vi "Proceed.vi"(7 "component is ready (Y)":bool=TRUE, 8 "error in (no error)":errorcluster, 10 "ProceedMessage":refnum<class "ProceedMessage.lvclass">, 11 "DAQOrcaFlash in":refnum<class "DAQOrcaFlash.lvclass">) -> (0 "error out":errorcluster, 2 "all observers are ready?":bool, 3 "DAQOrcaFlash out":refnum<class "DAQOrcaFlash.lvclass">)   [LabVIEW 2012, in "DAQOrcaFlash.lvclass"]
uses:
  DAQOrcaFlash.lvclass
  <vilib>/Distrio/Murmex/ProceedMessage/ProceedMessage.lvclass
  DAQOrcaFlash.lvclass/DAQOrcaFlash.ctl
  <vilib>/Distrio/Murmex/Murmex/Murmex.lvclass
panel:
  # "This method is called when the PROCEED\ntrigger is sent. \n\nOverride this method when your component needs to\nrespond to this trigger. \n\nCall parent for proper implementation"
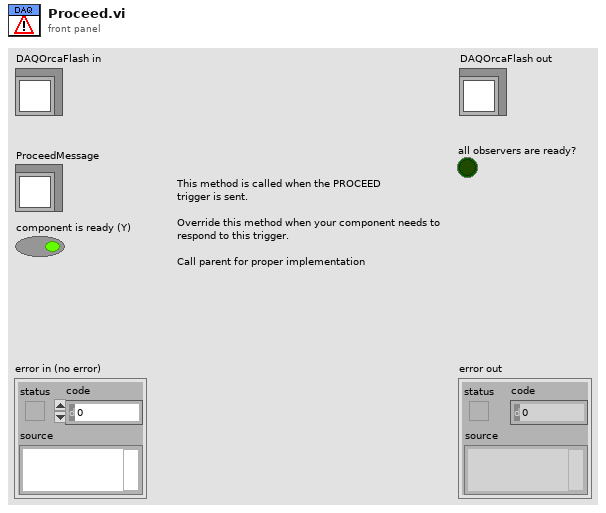
[diagram p1: front panel]
types:
  T1 = typedef "DAQOrcaFlash.lvclass/imaging_mode.ctl" = enum16{"focus mode", "single sweep"}
  T2 = typedef "IMAQ Image.ctl" = refnum<image>
  T3 = cluster{"width":u32, "height":u32, "datatype":u32}
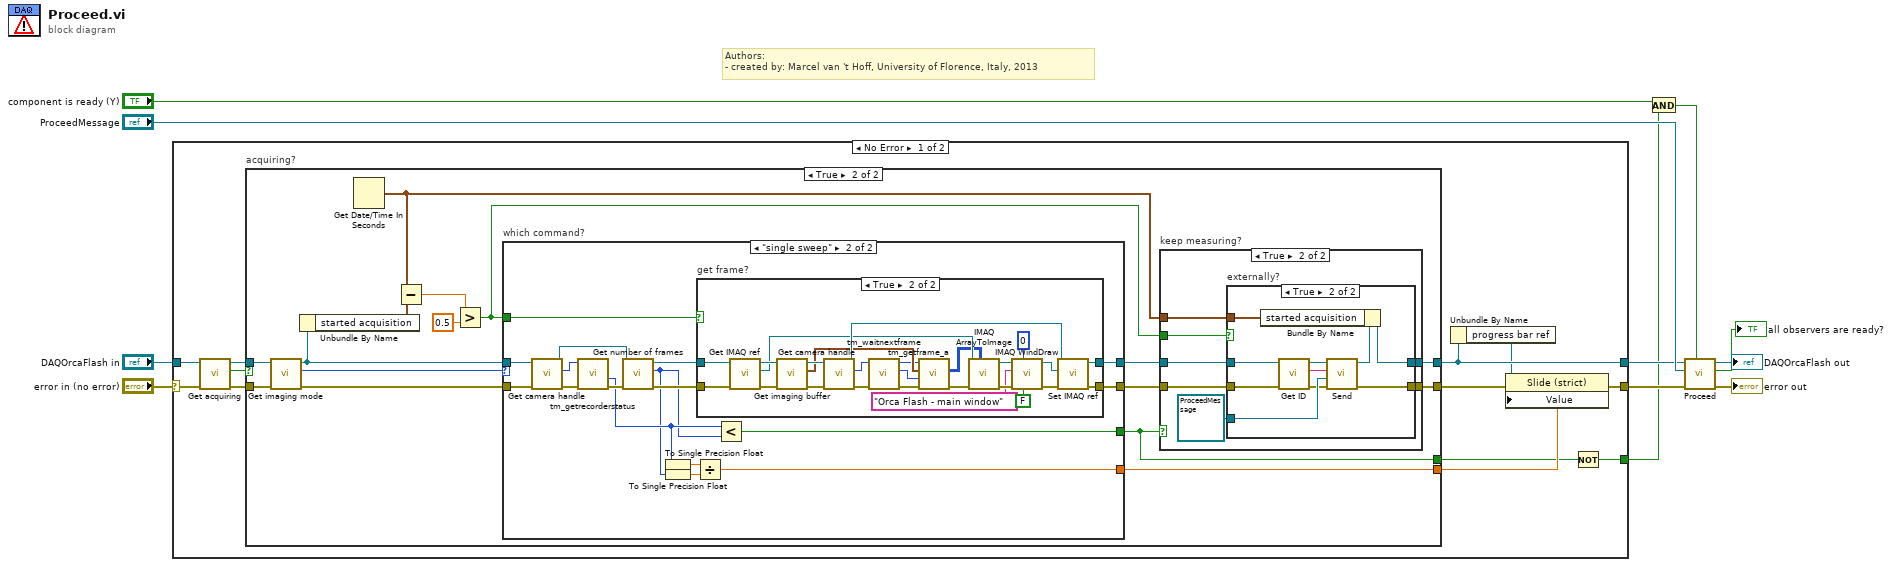
[diagram p0: block diagram]
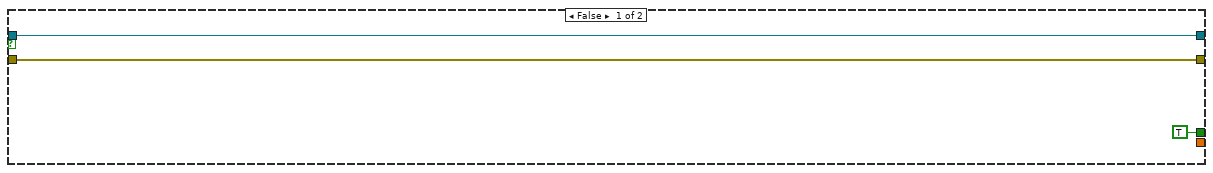
[diagram p2: hidden frame]
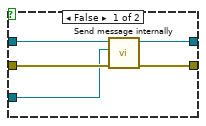
[diagram p4: hidden frame]
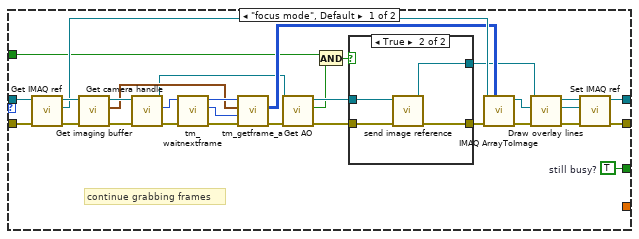
[diagram p5: hidden frame]
diagram:
  # "Authors: \n- created by: Marcel van 't Hoff, University of Florence, Italy, 2013"
  n1 = case shown="No Error" "error in (no error)" {
    selector: "error in (no error)" -> [w21 w149]
    tunnel: [w15 w149] -> w6
    tunnel: [w18 w148] -> w5
    tunnel: "DAQOrcaFlash in" -> [w23 w148]
    tunnel: [w12 _] -> w3
    frame No Error {
      n2 = call "Get acquiring.vi"("error in (no error)"=w21, "DAQMH121119OrcaFlash in"=w23) -> ("error out"=w20:errorcluster, "is acquiring?"=w19:bool, "DAQMH121119OrcaFlash out"=w22:refnum<class "DAQOrcaFlash.lvclass">)  [unwired: 7 in]
      n3 = case "acquiring?" shown="True" w19 {
        tunnel: [w25 w34] -> w14
        tunnel: [w26 w35] -> w18
        tunnel: w22 -> [w26 w40]
        tunnel: w20 -> [w25 w39]
        tunnel: [_ w38] -> w16
        tunnel: [TRUE ("proceed?") w27] -> w13
        frame False {
        }
        frame True {
          n4 = call "Get imaging mode.vi"("error in (no error)"=w39, "DAQMH121119OrcaFlash in"=w40) -> ("error out"=w42:errorcluster, "imaging mode"=w41:T1, "DAQMH121119OrcaFlash out"=w30:refnum<class "DAQOrcaFlash.lvclass">)  [unwired: 7 in]
          n5 = Unbundle By Name(w30) -> ("started acquisition"=w31:timestamp)
          n6 = Get Date/Time In Seconds() -> (seconds since 1Jan1904=w29:timestamp)
          n7 = Subtract(x=w29, y=w31) -> (x-y=w32:dbl)
          n8 = Greater?(x=w32, y=0.5) -> (0:w28:bool)
          n9 = case "which command?" shown="\"single sweep\"" w41 {
            tunnel: w42 -> [w96 w120]
            tunnel: w30 -> [w97 w118]
            tunnel: [w95 w108] -> w37
            tunnel: [w94 w109] -> w36
            tunnel: [_ w110] -> w38
            tunnel: [w93 w104] -> w27
            tunnel: w28 -> [w74 w107]
            frame "focus mode", Default {
              w93 = TRUE  # still busy?
              # "continue grabbing frames"
              n10 = call "Get IMAQ ref.vi"("error in (no error)"=w96, "DAQMH121119OrcaFlash in"=w97) -> ("error out"=w88:errorcluster, "IMAQ reference"=w82:T2, "DAQMH121119OrcaFlash out"=w90:refnum<class "DAQOrcaFlash.lvclass">)  [unwired: 7 in]
              n11 = call "Get imaging buffer.vi"("error in (no error)"=w88, "DAQMH121119OrcaFlash in"=w90) -> ("error out"=w87:errorcluster, "imaging buffer"=w84:T3, "DAQMH121119OrcaFlash out"=w89:refnum<class "DAQOrcaFlash.lvclass">)  [unwired: 5 in, 2 out]
              n12 = call "Get camera handle.vi"("error in (no error)"=w87, "DAQMH121119OrcaFlash in"=w89) -> ("error out"=w91:errorcluster, "cam handle"=w92:u32, "DAQMH121119OrcaFlash out"=w77:refnum<class "DAQOrcaFlash.lvclass">)  [unwired: 7 in]
              n13 = call <userlib>:"tm_waitnextframe.vi"("error in (no error)"=w91, "Handle in"=w92) -> ("error out"=w86:errorcluster, "Frame Index"=w83:i32, "Handle out"=w85:u32)  [unwired: 6 in, 1 out]
              n14 = call <userlib>:"tm_getframe_a.vi"("error in (no error)"=w86, "Frame Index"=w83, "Buffer"=w84, "Handle in"=w85) -> ("error out"=w79:errorcluster, "Data 16"=w80:u16[][])  [unwired: 3 in, 3 out]
              n15 = call-dynamic "Get AO.vi"("error in (no error)"=w79, "DAQOrcaFlash in"=w77) -> ("error out"=w78:errorcluster, "AO"=w75:bool, "DAQOrcaFlash out"=w76:refnum<class "DAQOrcaFlash.lvclass">)  [unwired: 7 in]
              n16 = And(x=w74, y=w75) -> (x .and. y?=w73:bool)
              n17 = case shown="True" w73 {
                tunnel: [w99 w101] -> w81
                tunnel: w78 -> [w99 w103]
                tunnel: w76 -> [w98 w102]
                tunnel: [w98 w100] -> w67
                frame False {
                }
                frame True {
                  n18 = call-dynamic "send image reference.vi"("error in (no error)"=w103, "DAQOrcaFlash in"=w102) -> ("error out"=w101:errorcluster, "DAQOrcaFlash out"=w100:refnum<class "DAQOrcaFlash.lvclass">)  [unwired: 8 in]
                }
              }
              n19 = call "IMAQ ArrayToImage"("Image Pixels (U16)"=w80, "error in (no error)"=w81, "Image"=w82) -> ("error out"=w72:errorcluster, "Image Out"=w70:T2)  [unwired: 7 in]
              n20 = call "Draw overlay lines.vi"("error in (no error)"=w72, "IMAQ reference"=w70, "DAQOrcaFlash in"=w67) -> ("error out"=w71:errorcluster, "IMAQ reference out"=w69:T2, "DAQOrcaFlash out"=w68:refnum<class "DAQOrcaFlash.lvclass">)  [unwired: 6 in]
              n21 = call "Set IMAQ ref.vi"("error in (no error)"=w71, "IMAQ reference"=w69, "DAQMH121119OrcaFlash in"=w68) -> ("error out"=w95:errorcluster, "DAQMH121119OrcaFlash out"=w94:refnum<class "DAQOrcaFlash.lvclass">)  [unwired: 7 in]
            }
            frame "single sweep" {
              n22 = call "Get camera handle.vi"("error in (no error)"=w120, "DAQMH121119OrcaFlash in"=w118) -> ("error out"=w119:errorcluster, "cam handle"=w117:u32, "DAQMH121119OrcaFlash out"=w116:refnum<class "DAQOrcaFlash.lvclass">)  [unwired: 7 in]
              n23 = call <userlib>:"tm_getrecorderstatus.vi"("error in (no error)"=w119, "Handle"=w117) -> ("error out"=w115:errorcluster, "Count"=w106:i32)  [unwired: 6 in, 2 out]
              n24 = call "Get number of frames.vi"("error in (no error)"=w115, "DAQMH121119OrcaFlash in"=w116) -> ("error out"=w114:errorcluster, "no. of frames"=w105:i32, "DAQMH121119OrcaFlash out"=w113:refnum<class "DAQOrcaFlash.lvclass">)  [unwired: 7 in]
              n25 = To Single Precision Float(number=w106) -> (single precision float=w111:sgl)
              n26 = To Single Precision Float(number=w105) -> (single precision float=w112:sgl)
              n27 = Divide(x=w111, y=w112) -> (x/y=w110:sgl)
              n28 = case "get frame?" shown="True" w107 {
                tunnel: w114 -> [w122 w139]
                tunnel: w113 -> [w121 w138]
                tunnel: [w121 w136] -> w109
                tunnel: [w122 w137] -> w108
                frame False {
                }
                frame True {
                  n29 = call "Get IMAQ ref.vi"("error in (no error)"=w139, "DAQMH121119OrcaFlash in"=w138) -> ("error out"=w146:errorcluster, "IMAQ reference"=w141:T2, "DAQMH121119OrcaFlash out"=w143:refnum<class "DAQOrcaFlash.lvclass">)  [unwired: 7 in]
                  n30 = call "Get imaging buffer.vi"("error in (no error)"=w146, "DAQMH121119OrcaFlash in"=w143) -> ("error out"=w147:errorcluster, "imaging buffer"=w135:T3, "DAQMH121119OrcaFlash out"=w145:refnum<class "DAQOrcaFlash.lvclass">)  [unwired: 5 in, 2 out]
                  n31 = call "Get camera handle.vi"("error in (no error)"=w147, "DAQMH121119OrcaFlash in"=w145) -> ("error out"=w131:errorcluster, "cam handle"=w134:u32, "DAQMH121119OrcaFlash out"=w144:refnum<class "DAQOrcaFlash.lvclass">)  [unwired: 7 in]
                  n32 = call <userlib>:"tm_waitnextframe.vi"("error in (no error)"=w131, "Handle in"=w134) -> ("error out"=w130:errorcluster, "Frame Index"=w132:i32, "Handle out"=w133:u32)  [unwired: 6 in, 1 out]
                  n33 = call <userlib>:"tm_getframe_a.vi"("error in (no error)"=w130, "Frame Index"=w132, "Buffer"=w135, "Handle in"=w133) -> ("error out"=w142:errorcluster, "Data 16"=w140:u16[][])  [unwired: 3 in, 3 out]
                  n34 = call "IMAQ ArrayToImage"("Image Pixels (U16)"=w140, "error in (no error)"=w142, "Image"=w141) -> ("error out"=w129:errorcluster, "Image Out"=w127:T2)  [unwired: 7 in]
                  n35 = call "IMAQ WindDraw"("Resize to Image Size? (Y)"=FALSE, "Window Number (0...15)"=0, "error in (no error)"=w129, "Title"="Orca Flash - main window", "Image"=w127) -> ("error out"=w128:errorcluster, "Image Out (duplicate)"=w126:T2)  [unwired: 5 in]
                  n36 = call "Set IMAQ ref.vi"("error in (no error)"=w128, "IMAQ reference"=w126, "DAQMH121119OrcaFlash in"=w144) -> ("error out"=w137:errorcluster, "DAQMH121119OrcaFlash out"=w136:refnum<class "DAQOrcaFlash.lvclass">)  [unwired: 7 in]
                }
              }
              n37 = Less?(x=w106, y=w105) -> (x < y?=w104:bool)
            }
          }
          n38 = case "keep measuring?" shown="True" w27 {
            tunnel: w37 -> [w43 w46]
            tunnel: [w43 w49] -> w34
            tunnel: w36 -> [w44 w51]
            tunnel: [w44 w50] -> w35
            tunnel: w28 -> [_ w48]
            tunnel: w29 -> [_ w47]
            frame False {
            }
            frame True {
              n39 = case "externally?" shown="True" w48 {
                tunnel: w46 -> [w56 w62]
                tunnel: refnum<class "ProceedMessage.lvclass"> refnum ("ProceedMessage") -> [w55 w64]
                tunnel: w51 -> [w54 w65]
                tunnel: [w53 w57] -> w50
                tunnel: [w52 w66] -> w49
                tunnel: w47 -> [_ w59]
                frame False {
                  n40 = call <vilib>:"Send message internally.vi"("error in (no error)"=w56, "Message"=w55, "Murmex in"=w54) -> ("error out"=w52:errorcluster, "Murmex out"=w53:refnum<class "DAQOrcaFlash.lvclass">)  [unwired: 7 in]
                }
                frame True {
                  n41 = call <vilib>:"Get ID.vi"("error in (no error)"=w62, "Murmex in"=w65) -> ("error out"=w61:errorcluster, "component id"=w60:string, "Murmex out"=w63:refnum<class "DAQOrcaFlash.lvclass">)  [unwired: 7 in]
                  n42 = call <vilib>:"Send.vi"("error in (no error)"=w61, "Message"=w64, "recipient"=w60, "Murmex in"=w63) -> ("error out"=w66:errorcluster, "Murmex out"=w58:refnum<class "DAQOrcaFlash.lvclass">)  [unwired: 6 in]
                  n43 = Bundle By Name(cluster=w58, "started acquisition"=w59) -> (w57:refnum<class "DAQOrcaFlash.lvclass">)
                }
              }
            }
          }
        }
      }
      n44 = Unbundle By Name(w18) -> ("progress bar ref"=w17:refnum<vi>)
      n45 = property class="Slide (strict)"(reference=w17, error in=w14, "Value"=w16) -> (error out=w15:errorcluster)  [unwired: 1 out]
      n46 = Not(x=w13) -> (.not. x?=w12:bool)
    }
    frame Error {
    }
  }
  n47 = And(x="component is ready (Y)", y=w3) -> (x .and. y?=w2:bool)
  n48 = call-parent "Proceed.vi"("component is ready (Y)"=w2, "error in (no error)"=w6, "ProceedMessage"="ProceedMessage", "Murmex in"=w5) -> ("error out"=→"error out":errorcluster, "all observers are ready?"=→"all observers are ready?":bool, "Murmex out"=→"DAQOrcaFlash out":refnum<class "DAQOrcaFlash.lvclass">)  [unwired: 5 in]
